vi "convert_int32Array_to_string.vi"(2 "Max Elements Count (All)":i32=-1, 4 "I32 array in":i32[](array[numeric]), 5 "String to add before (\"\")":string) -> (1 "string out":string)   [LabVIEW 2020, in "Rohde&Schwarz RTx Oscilloscopes.lvlib" / "rsidr_core.lvlib"]
uses:
  rsidr_core.lvlib
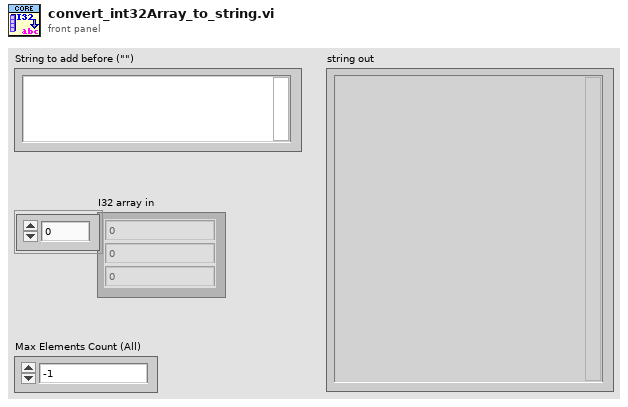
[diagram p1: front panel]
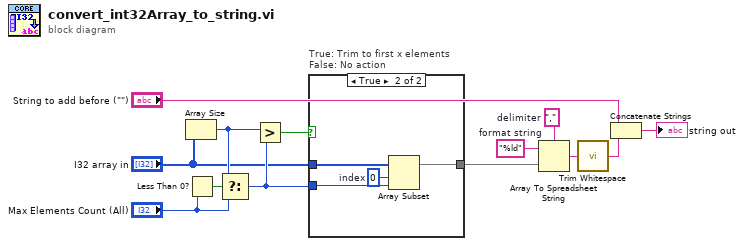
[diagram p0: block diagram]
diagram:
  w10 = "%ld"  # format string
  w13 = ","  # delimiter
  n1 = Array Size(array="I32 array in") -> (size(s)=w8:i32)
  n2 = Less Than 0?(x="Max Elements Count (All)") -> (x < 0?=w9:bool)
  n3 = Select(t=w8, s=w9, f="Max Elements Count (All)") -> (s? t:f=w6:i32)
  n4 = Greater?(x=w8, y=w6) -> (0:w7:bool)
  n5 = case "True: Trim to first x elements\nFalse: No action" shown="True" w7 {
    tunnel: [w14 w15] -> w5
    tunnel: "I32 array in" -> [w14 w18]
    tunnel: w6 -> [_ w16]
    frame False {
    }
    frame True {
      w17 = 0  # index
      n6 = Array Subset(array=w18, index=w17, length=w16) -> (w15:i32[])
    }
  }
  n7 = Array To Spreadsheet String(delimiter (Tab)=w13, array=w5, 3:w10) -> (spreadsheet string=w12:string)
  n8 = call "Trim Whitespace.vi"("string"=w12) -> ("trimmed string"=w11:string)  [unwired: 1 in]
  n9 = Concatenate Strings("String to add before (\"\")", w11) -> (→"string out":string)
